vi "FPGA Watchdog - Elapsed Time.vi"(7 "Reset":bool, 10 "Timeout Period":u64, 11 "Current Time":u32) -> (2 "Timeout":bool, 3 "Elapsed Time":u64)   [LabVIEW 2013]
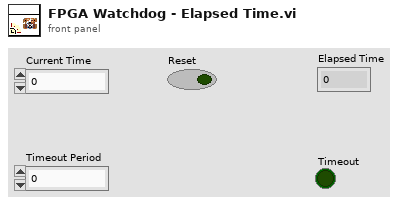
[diagram p1: front panel]
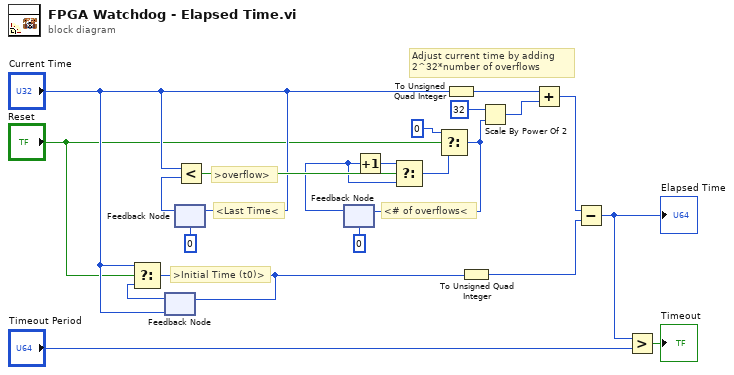
[diagram p0: block diagram]
diagram:
  # "Adjust current time by adding 2^32*number of overflows"
  # "<# of overflows<"
  # ">Initial Time (t0)>"
  # "<Last Time<"
  # ">overflow>"
  n1 = feedback #1("Current Time") -> (w9:u32)
  n2 = Select(t="Current Time", s="Reset", f=w9) -> (s? t:f=w7:u32)
  n3 = feedback-in #1(w7) -> ()
  n4 = feedback-in #2("Current Time") -> ()
  n5 = feedback #2(u32 0 ("unsigned 64bit integer")) -> (w14:u32)
  n6 = Less?(x="Current Time", y=w14) -> (x < y?=w12:bool)
  n7 = feedback #3(u64 0 ("unsigned 64bit integer")) -> (w4:u64)
  n8 = Increment(x=w4) -> (x+1=w11:u64)
  n9 = Select(t=w11, s=w12, f=w4) -> (s? t:f=w3:u64)
  n10 = Select(t=u64 0 ("unsigned 64bit integer"), s="Reset", f=w3) -> (s? t:f=w1:u64)
  n11 = feedback-in #3(w1) -> ()
  n12 = To Unsigned Quad Integer(1:"Current Time") -> (0:w13:u64)
  n13 = To Unsigned Quad Integer(1:w7) -> (0:w6:u64)
  n14 = Scale By Power Of 2(n=32, x=w1) -> (x*2^n=w17:u64)
  n15 = Add(x=w13, y=w17) -> (x+y=w8:u64)
  n16 = Subtract(x=w8, y=w6) -> (x-y=w5:u64)
  "Elapsed Time" <- w5
  n17 = Greater?(x=w5, y="Timeout Period") -> (0:→"Timeout":bool)
